vi "Chebyshev Filter PtByPt.vi"(4 "order":i32=2, 5 "initialize":bool, 6 "ripple(dB)":dbl=0.1 format="%0.2f", 7 "filter type":T1, 8 "low cutoff freq: fl":dbl=0.125 format="%0.3f", 9 "high cutoff freq: fh":dbl=0.45000000000000007 format="%0.3f", 10 "sampling freq: fs":dbl=1.0 format="%0.2f", 11 "x":dbl format="%0.2f") -> (0 "error":i32, 3 "Filtered x":dbl format="%0.2f")   [LabVIEW 2020, in "NI_PtbyPt.lvlib"]
doc: "Generates a digital Chebyshev filter by calling the Chebyshev Coefficients VI."
uses:
  NI_PtbyPt.lvlib
  Filter Passband Type.ctl
  NI_AALBase.lvlib
panel:
  # "PbP_Butterworth Filter"
  # "Filter Controls"
  # "Frequency Controls"
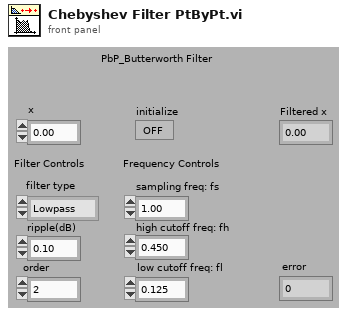
[diagram p1: front panel]
types:
  T1 = typedef "NI_AALBase.lvlib/Filter Passband Type.ctl" = enum32{"Lowpass", "Highpass", "Bandpass", "Bandstop"}
  T2 = cluster{"filter structure":enum32{"IIR 2nd Order", "IIR 4th Order"}, "Reverse Coefficients":dbl[], "Forward Coefficients":dbl[]}
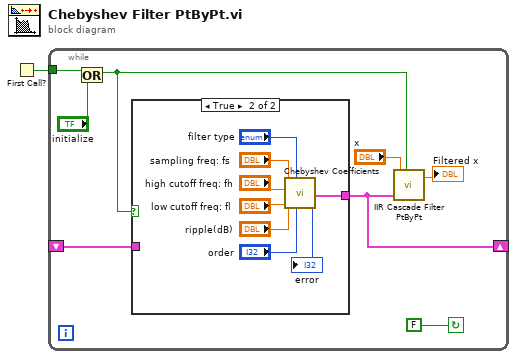
[diagram p0: block diagram]
diagram:
  n1 = First Call?() -> (First Call?: T/F=w1:bool)
  n2 = while {
    tunnel: w1 -> [w4]
    shift-left: _ -> [w8]
    shift-right: [w6] -> _
    stop <- FALSE continue-if-true
    n3 = Or(x=w4, y="initialize") -> (x .or. y?=w2:bool)
    n4 = case shown="True" w2 {
      tunnel: [w10 w12] -> w6
      tunnel: w8 -> [w10 _]
      frame False {
      }
      frame True {
        n5 = call "Chebyshev Coefficients.vi"("order"="order", "filter type"="filter type", "ripple(dB)"="ripple(dB)", "low cutoff freq: fl"="low cutoff freq: fl", "high cutoff freq: fh"="high cutoff freq: fh", "sampling freq: fs"="sampling freq: fs") -> ("error"=→"error":i32, "IIR Filter Cluster"=w12:T2)  [unwired: 4 in]
      }
    }
    n6 = call "IIR Cascade Filter PtByPt.vi"("initialize"=w2, "IIR Filter Cluster"=w6, "x"="x") -> ("Filtered x"=→"Filtered x":dbl)  [unwired: 2 out]
  }
